vi "GT Get Crd Vel.vi"(8 "error in (no error)":errorcluster caption="错误输入（无错误）", 9 "pSynVel":dbl, 10 "crd":i16, 11 "cardNum":i16) -> (0 "error out":errorcluster caption="错误输出", 1 "pSynVel out":dbl, 3 "function return":i16)   [LabVIEW 2020, in "gts.lvlib"]
doc: "GT_API GT_GetCrdVel(short cardNum,short crd,double *pSynVel);"
uses:
  gts.lvlib
  dll/32bit/multi_card/gts.dll
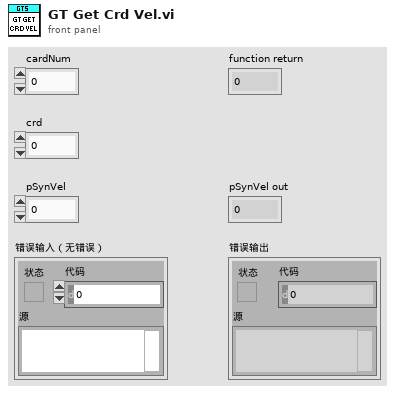
[diagram p1: front panel]
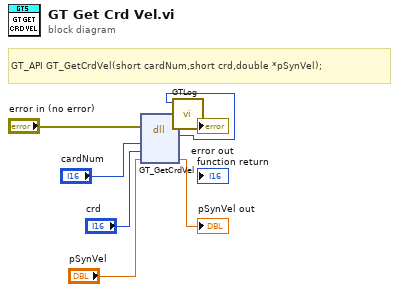
[diagram p0: block diagram]
diagram:
  # "GT_API GT_GetCrdVel(short cardNum,short crd,double *pSynVel);"
  n1 = dll-call lib="C:/1228/dll/32bit/multi_card/gts.dll" fn="GT_GetCrdVel"(error in="error in (no error)", "cardNum"="cardNum", "crd"="crd", "pSynVel"="pSynVel") -> (error out=w3:errorcluster, w1:i16, "pSynVel"=→"pSynVel out":dbl)  [unwired: 4 in, 1 out]
  n2 = call "GTLog.vi"("error in (no error)"=w3, "Numeric"=w1) -> ("error out"=→"error out":errorcluster)  [unwired: 9 in]
